vi "Extract Number From Quotes.vi"(1 "Array of Results":string[](array[string])) -> (0 "Numeric":dbl)   [LabVIEW 2013]
doc: "This VI extracts a number that is in quotes from a result array."
uses:
  <vilib>/regexp/Match Regular Expression.xnode
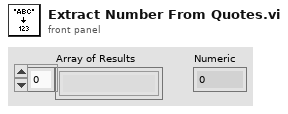
[diagram p1: front panel]
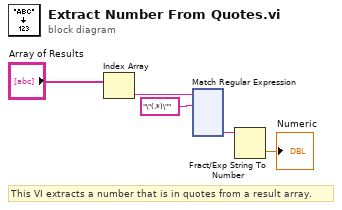
[diagram p0: block diagram]
diagram:
  # "This VI extracts a number that is in quotes from a result array."
  n1 = Index Array(array="Array of Results") -> (element=w3:string)  [unwired: 1 in]
  n2 = xnode "Match Regular Expression"("input string"=w3, "regular expression"="\"(.*)\"") -> ("submatch 1"=w4:string)  [unwired: 4 in, 5 out]
  n3 = Fract/Exp String To Number(string=w4) -> (number=→"Numeric":dbl)  [unwired: 3 in, 1 out]
